vi "Add Employees Info to Employee Table.vi"(8 "error in (no error)":errorcluster caption="错误输入（无错误）", 10 "Employees Info":T1[](array[typedef]), 11 "Employee 输入":refnum<class "Employee.lvclass"> caption="DNL_LabVIEW Object in") -> (0 "error out":errorcluster caption="错误输出", 3 "Employee 输出":refnum<class "Employee.lvclass"> caption="DNL_LabVIEW Object out")   [LabVIEW 2012, in "Employee.lvclass"]
uses:
  Employee.lvclass
  Custom Def/Employee Info.ctl
  Employee.lvclass/Employee.ctl
  Data Table/DataTable.lvclass
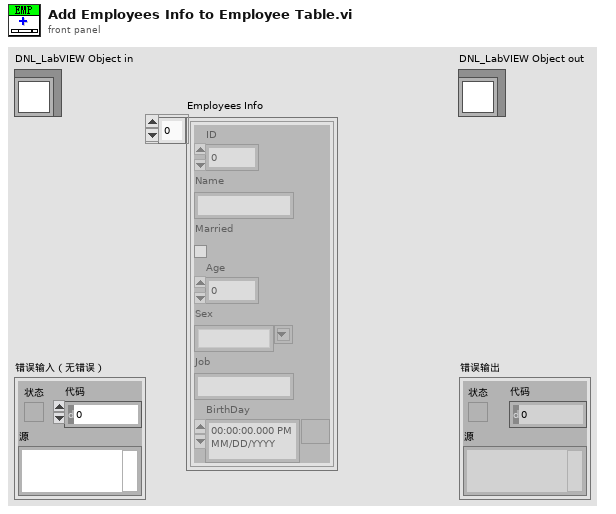
[diagram p1: front panel]
types:
  T1 = typedef "Employee Info.ctl" = cluster{"ID":u16, "Name":string, "Married":bool, "Age":u8, "Sex":string, "Job":string, "BirthDay":timestamp}
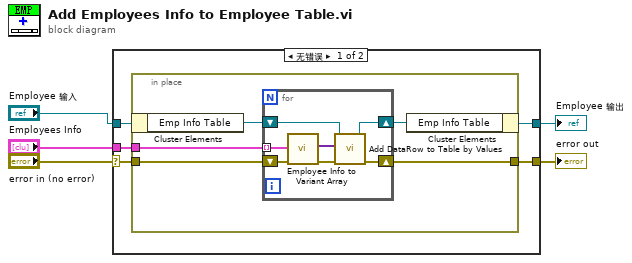
[diagram p0: block diagram]
diagram:
  n1 = case shown="无错误" "error in (no error)" {
    selector: "error in (no error)" -> [w8 w24]
    tunnel: [w7 w24] -> w4
    tunnel: [w6 w23] -> w2
    tunnel: "Employee 输入" -> [w10 w23]
    tunnel: "Employees Info" -> [w9 _]
    frame No Error {
      n2 = in-place {
        in-place-border: w9 -> [w15]
        in-place-border: w8 -> [w12]
        in-place-border: [w11] -> w7
        n3 = in-place-cluster #1(w10) -> ("Emp Info Table"=w14:refnum<class "DataTable.lvclass">)
        n4 = for {
          tunnel: w15 -> [w19] mode=indexing
          shift-right: [w21] -> w13
          shift-left: w14 -> [w22]
          shift-right: [w20] -> w11
          shift-left: w12 -> [w18]
          n5 = call "Employee Info to Variant Array.vi"("error in (no error)"=w18, "Employee Info"=w19) -> ("error out"=w17:errorcluster, "Employee Info Var Array"=w16:variant[])  [unwired: 7 in, 1 out]
          n6 = call "Add DataRow to Table by Values.vi"("error in (no error)"=w17, "values"=w16, "DataTable 输入"=w22) -> ("error out"=w20:errorcluster, "DataTable 输出"=w21:refnum<class "DataTable.lvclass">)  [unwired: 7 in]
        }
        n7 = in-place-cluster #1("Emp Info Table"=w13) -> (w6:refnum<class "Employee.lvclass">)
      }
    }
    frame Error {
    }
  }
  "error out" <- w4
  "Employee 输出" <- w2
